vi "FT10_PXI-2565 Tester.vi"() -> ()   [LabVIEW 2024]
uses:
  <instrlib>/niSwitch/niSwitch.llb/niSwitch Topologies.ctl
  Controls/QMH Fundamentals - Message Cluster.ctl
  <instrlib>/niSwitch/niSwitch.llb/niSwitch Connect Channels (Single).vi
  <instrlib>/niSwitch/niSwitch.llb/niSwitch Disconnect Channels (Single).vi
panel:
  in  "Stop":bool
  out "instrument handle out":refnum<k15>
  out "error out":errorcluster {"code" format="%.0x"}
  in  "error in (no error)":errorcluster {"code" format="%.0x"}
  in  "reset device (boolean value)":bool=TRUE
  in  "simulate (boolean value)":bool
  in  "resource name":refnum<k15>="PXI1Slot7"
  in  "topology name":T1="2565/16-SPST"
  in  "Tab Control":enum32{"Manual", "Named"}(tab)
  in  "Channel 1":string
  in  "Channel 2":string
  in  "Disconnect - Manual":bool
  in  "Connect - Manual":bool
  in  "Enum":T2(ring)
  in  "Connect - Named":bool
  in  "Disconnect - Named":bool
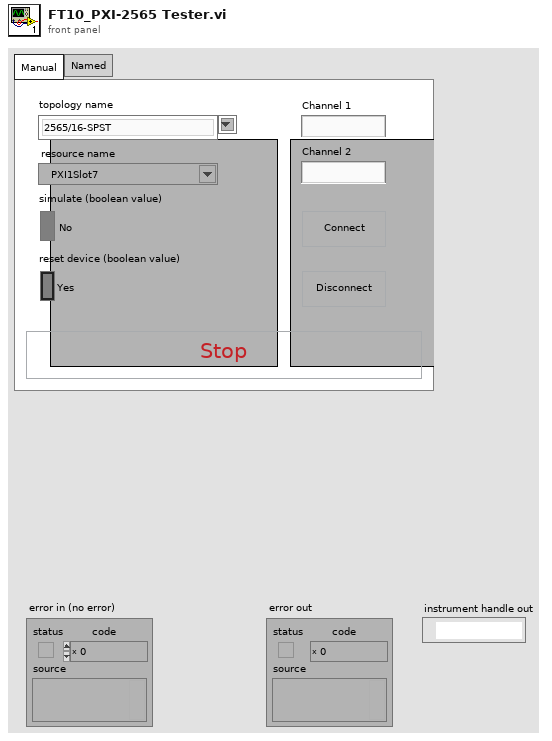
[diagram p1: front panel]
types:
  T1 = typedef "niSwitch Topologies.ctl" = string
  T2 = enum16{"Mono1 - Coag", "Mono1 - Cut", "Mono2 - Coag", "Mono2 - Cut", "Mono2 - Valleylab", "Mono2 - Spare", "Bipolar - Bipolar", "Advanced - Bipolar", "Advanced - Seal", "Advanced - Cut", "Advanced - Coag", "Advanced - Spare"}
  T3 = typedef "QMH Fundamentals - Message Cluster.ctl" = cluster{"Message":string, "Message Data":variant}
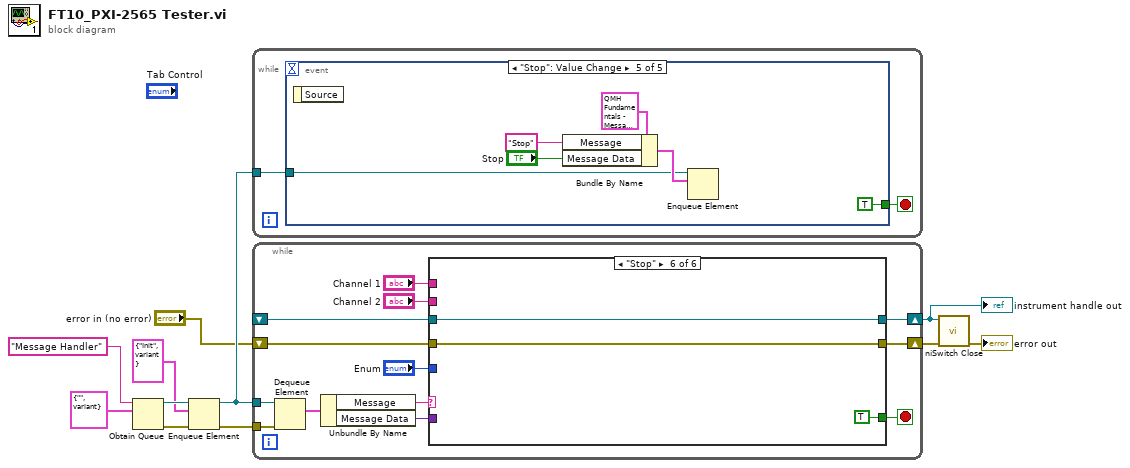
[diagram p0: block diagram]
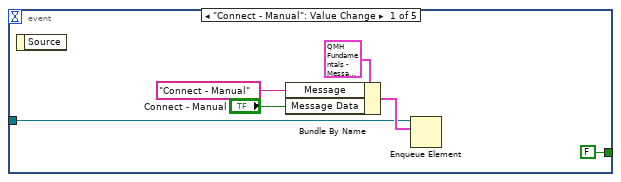
[diagram p2: hidden frame]
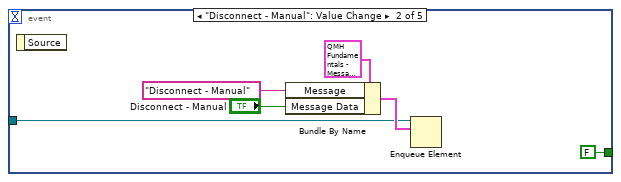
[diagram p3: hidden frame]
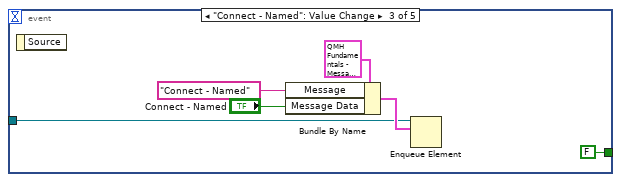
[diagram p4: hidden frame]
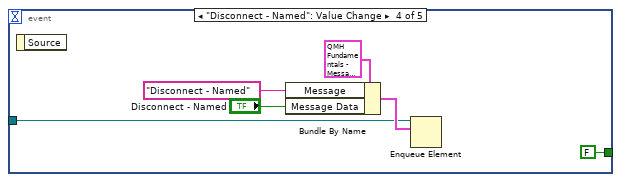
[diagram p5: hidden frame]
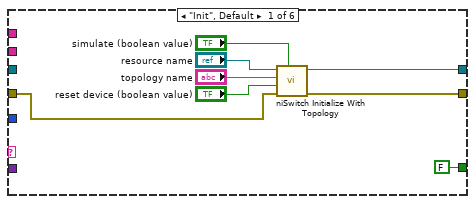
[diagram p6: hidden frame]
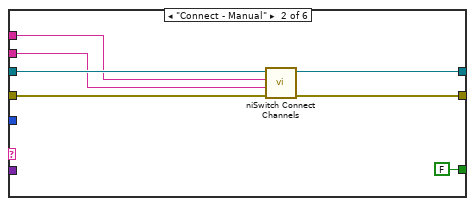
[diagram p7: hidden frame]
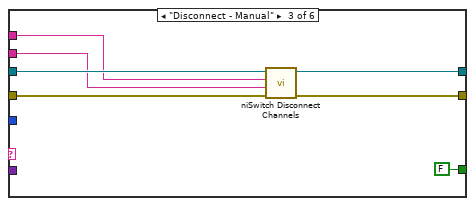
[diagram p8: hidden frame]
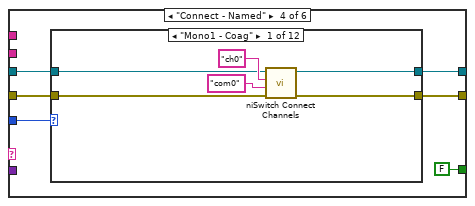
[diagram p9: hidden frame]
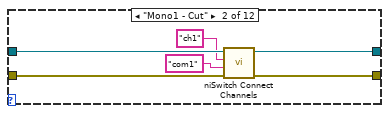
[diagram p10: hidden frame]
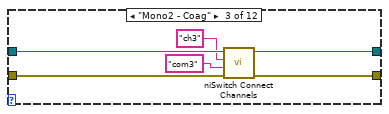
[diagram p11: hidden frame]
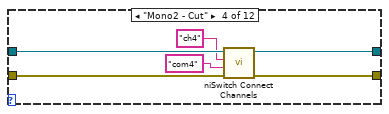
[diagram p12: hidden frame]
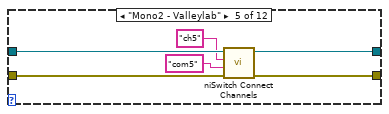
[diagram p13: hidden frame]
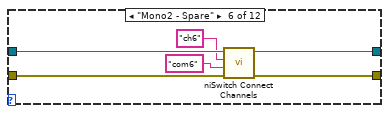
[diagram p14: hidden frame]
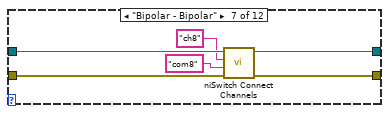
[diagram p15: hidden frame]
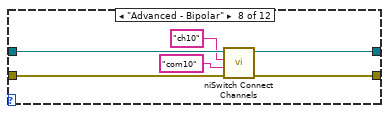
[diagram p16: hidden frame]
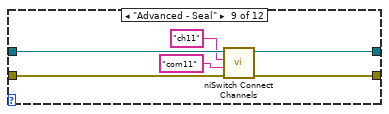
[diagram p17: hidden frame]
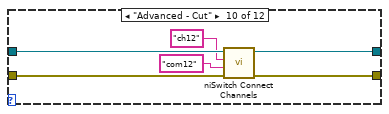
[diagram p18: hidden frame]
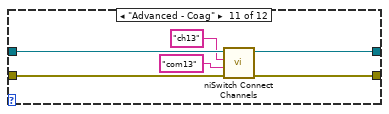
[diagram p19: hidden frame]
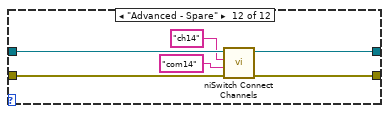
[diagram p20: hidden frame]
diagram:
  n1 = Obtain Queue(name (unnamed)="Message Handler", element data type=T3 {"Message"="", "Message Data"=variant} ("Message Cluster")) -> (queue out=w9:refnum<queue>, error out=w10:errorcluster)  [unwired: 3 in, 1 out]
  n2 = Enqueue Element(queue=w9, element=T3 {"Message"="Init", "Message Data"=variant}, error in (no error)=w10) -> (queue out=w5:refnum<queue>, error out=w6:errorcluster)  [unwired: 1 in, 1 out]
  n3 = while {
    tunnel: w5 -> [w13]
    stop <- w12 stop-if-true
    n4 = event shown="[4] \"Stop\": Value Change" {
      selector: _ -> [_ _ _ _ _]
      dyn-events: _ -> [_ _ _ _ _]
      timeout: _ -> [_ _ _ _ _]
      tunnel: w13 -> [w15 w22 w28 w34 w40]
      tunnel: [FALSE FALSE FALSE FALSE TRUE] -> w12
      event "Connect - Manual": Value Change {
        n5 = event-data() -> ()  [unwired: 1 in, 1 out]
        n6 = Bundle By Name(cluster=T3 {"Message"="Fornax Connect/Disconnect", "Message Data"=variant} ("element"), "Message"="Connect - Manual", "Message Data"="Connect - Manual") -> (w19:T3)
        n7 = Enqueue Element(queue=w15, element=w19) -> ()  [unwired: 2 in, 3 out]
      }
      event "Disconnect - Manual": Value Change {
        n8 = event-data() -> ()  [unwired: 1 in, 1 out]
        n9 = Bundle By Name(cluster=T3 {"Message"="Fornax Connect/Disconnect", "Message Data"=variant} ("element"), "Message"="Disconnect - Manual", "Message Data"="Disconnect - Manual") -> (w25:T3)
        n10 = Enqueue Element(queue=w22, element=w25) -> ()  [unwired: 2 in, 3 out]
      }
      event "Connect - Named": Value Change {
        n11 = event-data() -> ()  [unwired: 1 in, 1 out]
        n12 = Bundle By Name(cluster=T3 {"Message"="Fornax Connect/Disconnect", "Message Data"=variant} ("element"), "Message"="Connect - Named", "Message Data"="Connect - Named") -> (w31:T3)
        n13 = Enqueue Element(queue=w28, element=w31) -> ()  [unwired: 2 in, 3 out]
      }
      event "Disconnect - Named": Value Change {
        n14 = event-data() -> ()  [unwired: 1 in, 1 out]
        n15 = Bundle By Name(cluster=T3 {"Message"="Fornax Connect/Disconnect", "Message Data"=variant} ("element"), "Message"="Disconnect - Named", "Message Data"="Disconnect - Named") -> (w37:T3)
        n16 = Enqueue Element(queue=w34, element=w37) -> ()  [unwired: 2 in, 3 out]
      }
      event "Stop": Value Change {
        n17 = event-data() -> ()  [unwired: 1 in, 1 out]
        n18 = Bundle By Name(cluster=T3 {"Message"="Fornax Connect/Disconnect", "Message Data"=variant} ("element"), "Message"="Stop", "Message Data"="Stop") -> (w43:T3)
        n19 = Enqueue Element(queue=w40, element=w43) -> ()  [unwired: 2 in, 3 out]
      }
    }
  }
  n20 = while {
    tunnel: w5 -> [w55]
    tunnel: w6 -> [w54]
    shift-right: [w51] -> w3
    shift-left: _ -> [w50]
    shift-right: [w47] -> w2
    shift-left: "error in (no error)" -> [w46]
    stop <- w44 stop-if-true
    n21 = Dequeue Element(queue=w55, error in (no error)=w54) -> (element=w56:T3)  [unwired: 1 in, 3 out]
    n22 = Unbundle By Name(w56) -> ("Message"=w53:string, "Message Data"=w52:variant)
    n23 = case shown="\"Stop\"" w53 {
      tunnel: w52 -> [_ _ _ _ _ _]
      tunnel: [w60 w68 w73 w82 w160 w237] -> w51
      tunnel: w50 -> [_ w71 w78 w84 w162 w237]
      tunnel: "Channel 1" -> [_ w70 w77 _ _ _]
      tunnel: "Channel 2" -> [_ w69 w76 _ _ _]
      tunnel: [w59 w66 w74 w81 w159 w236] -> w47
      tunnel: w46 -> [w58 w67 w75 w83 w161 w236]
      tunnel: "Enum" -> [_ _ _ w80 w158 _]
      tunnel: [FALSE FALSE FALSE FALSE FALSE TRUE] -> w44
      frame "Init", Default {
        n24 = call <instrlib>:"niSwitch Initialize With Topology.vi"("simulate (boolean value)"="simulate (boolean value)", "error in (no error)"=w58, "reset device (boolean value)"="reset device (boolean value)", "topology name"="topology name", "resource name"="resource name") -> ("error out"=w59:errorcluster, "instrument handle out"=w60:refnum<k15>)  [unwired: 5 in]
      }
      frame "Connect - Manual" {
        n25 = call-poly <instrlib>:"niSwitch Connect Channels.vi"("error in (no error)"=w67, "channel 2"=w69, "channel 1"=w70, "instrument handle"=w71) -> ("error out"=w66:errorcluster, "instrument handle out"=w68:refnum<k15>)  [unwired: 6 in]
      }
      frame "Disconnect - Manual" {
        n26 = call-poly <instrlib>:"niSwitch Disconnect Channels.vi"("error in (no error)"=w75, "channel 2"=w76, "channel 1"=w77, "instrument handle"=w78) -> ("error out"=w74:errorcluster, "instrument handle out"=w73:refnum<k15>)  [unwired: 6 in]
      }
      frame "Connect - Named" {
        n27 = case shown="\"Mono1 - Coag\"" w80 {
          tunnel: w84 -> [w88 w96 w102 w108 w114 w120 w126 w132 w138 w144 w150 w156]
          tunnel: w83 -> [w87 w95 w101 w107 w113 w119 w125 w131 w137 w143 w149 w155]
          tunnel: [w86 w94 w100 w106 w112 w118 w124 w130 w136 w142 w148 w154] -> w82
          tunnel: [w85 w93 w99 w105 w111 w117 w123 w129 w135 w141 w147 w153] -> w81
          frame "Mono1 - Coag" {
            n28 = call-poly <instrlib>:"niSwitch Connect Channels.vi"("error in (no error)"=w87, "channel 2"="com0", "channel 1"="ch0", "instrument handle"=w88) -> ("error out"=w85:errorcluster, "instrument handle out"=w86:refnum<k15>)  [unwired: 6 in]
          }
          frame "Mono1 - Cut" {
            n29 = call-poly <instrlib>:"niSwitch Connect Channels.vi"("error in (no error)"=w95, "channel 2"="com1", "channel 1"="ch1", "instrument handle"=w96) -> ("error out"=w93:errorcluster, "instrument handle out"=w94:refnum<k15>)  [unwired: 6 in]
          }
          frame "Mono2 - Coag" {
            n30 = call-poly <instrlib>:"niSwitch Connect Channels.vi"("error in (no error)"=w101, "channel 2"="com3", "channel 1"="ch3", "instrument handle"=w102) -> ("error out"=w99:errorcluster, "instrument handle out"=w100:refnum<k15>)  [unwired: 6 in]
          }
          frame "Mono2 - Cut" {
            n31 = call-poly <instrlib>:"niSwitch Connect Channels.vi"("error in (no error)"=w107, "channel 2"="com4", "channel 1"="ch4", "instrument handle"=w108) -> ("error out"=w105:errorcluster, "instrument handle out"=w106:refnum<k15>)  [unwired: 6 in]
          }
          frame "Mono2 - Valleylab" {
            n32 = call-poly <instrlib>:"niSwitch Connect Channels.vi"("error in (no error)"=w113, "channel 2"="com5", "channel 1"="ch5", "instrument handle"=w114) -> ("error out"=w111:errorcluster, "instrument handle out"=w112:refnum<k15>)  [unwired: 6 in]
          }
          frame "Mono2 - Spare" {
            n33 = call-poly <instrlib>:"niSwitch Connect Channels.vi"("error in (no error)"=w119, "channel 2"="com6", "channel 1"="ch6", "instrument handle"=w120) -> ("error out"=w117:errorcluster, "instrument handle out"=w118:refnum<k15>)  [unwired: 6 in]
          }
          frame "Bipolar - Bipolar" {
            n34 = call-poly <instrlib>:"niSwitch Connect Channels.vi"("error in (no error)"=w125, "channel 2"="com8", "channel 1"="ch8", "instrument handle"=w126) -> ("error out"=w123:errorcluster, "instrument handle out"=w124:refnum<k15>)  [unwired: 6 in]
          }
          frame "Advanced - Bipolar" {
            n35 = call-poly <instrlib>:"niSwitch Connect Channels.vi"("error in (no error)"=w131, "channel 2"="com10", "channel 1"="ch10", "instrument handle"=w132) -> ("error out"=w129:errorcluster, "instrument handle out"=w130:refnum<k15>)  [unwired: 6 in]
          }
          frame "Advanced - Seal" {
            n36 = call-poly <instrlib>:"niSwitch Connect Channels.vi"("error in (no error)"=w137, "channel 2"="com11", "channel 1"="ch11", "instrument handle"=w138) -> ("error out"=w135:errorcluster, "instrument handle out"=w136:refnum<k15>)  [unwired: 6 in]
          }
          frame "Advanced - Cut" {
            n37 = call-poly <instrlib>:"niSwitch Connect Channels.vi"("error in (no error)"=w143, "channel 2"="com12", "channel 1"="ch12", "instrument handle"=w144) -> ("error out"=w141:errorcluster, "instrument handle out"=w142:refnum<k15>)  [unwired: 6 in]
          }
          frame "Advanced - Coag" {
            n38 = call-poly <instrlib>:"niSwitch Connect Channels.vi"("error in (no error)"=w149, "channel 2"="com13", "channel 1"="ch13", "instrument handle"=w150) -> ("error out"=w147:errorcluster, "instrument handle out"=w148:refnum<k15>)  [unwired: 6 in]
          }
          frame "Advanced - Spare" {
            n39 = call-poly <instrlib>:"niSwitch Connect Channels.vi"("error in (no error)"=w155, "channel 2"="com14", "channel 1"="ch14", "instrument handle"=w156) -> ("error out"=w153:errorcluster, "instrument handle out"=w154:refnum<k15>)  [unwired: 6 in]
          }
        }
      }
      frame "Disconnect - Named" {
        n40 = case shown="\"Mono1 - Coag\"" w158 {
          tunnel: w162 -> [w166 w174 w180 w186 w192 w198 w204 w210 w216 w222 w228 w234]
          tunnel: w161 -> [w165 w173 w179 w185 w191 w197 w203 w209 w215 w221 w227 w233]
          tunnel: [w164 w172 w178 w184 w190 w196 w202 w208 w214 w220 w226 w232] -> w160
          tunnel: [w163 w171 w177 w183 w189 w195 w201 w207 w213 w219 w225 w231] -> w159
          frame "Mono1 - Coag" {
            n41 = call-poly <instrlib>:"niSwitch Disconnect Channels.vi"("error in (no error)"=w165, "channel 2"="com0", "channel 1"="ch0", "instrument handle"=w166) -> ("error out"=w163:errorcluster, "instrument handle out"=w164:refnum<k15>)  [unwired: 6 in]
          }
          frame "Mono1 - Cut" {
            n42 = call-poly <instrlib>:"niSwitch Disconnect Channels.vi"("error in (no error)"=w173, "channel 2"="com1", "channel 1"="ch1", "instrument handle"=w174) -> ("error out"=w171:errorcluster, "instrument handle out"=w172:refnum<k15>)  [unwired: 6 in]
          }
          frame "Mono2 - Coag" {
            n43 = call-poly <instrlib>:"niSwitch Disconnect Channels.vi"("error in (no error)"=w179, "channel 2"="com3", "channel 1"="ch3", "instrument handle"=w180) -> ("error out"=w177:errorcluster, "instrument handle out"=w178:refnum<k15>)  [unwired: 6 in]
          }
          frame "Mono2 - Cut" {
            n44 = call-poly <instrlib>:"niSwitch Disconnect Channels.vi"("error in (no error)"=w185, "channel 2"="com4", "channel 1"="ch4", "instrument handle"=w186) -> ("error out"=w183:errorcluster, "instrument handle out"=w184:refnum<k15>)  [unwired: 6 in]
          }
          frame "Mono2 - Valleylab" {
            n45 = call-poly <instrlib>:"niSwitch Disconnect Channels.vi"("error in (no error)"=w191, "channel 2"="com5", "channel 1"="ch5", "instrument handle"=w192) -> ("error out"=w189:errorcluster, "instrument handle out"=w190:refnum<k15>)  [unwired: 6 in]
          }
          frame "Mono2 - Spare" {
            n46 = call-poly <instrlib>:"niSwitch Disconnect Channels.vi"("error in (no error)"=w197, "channel 2"="com6", "channel 1"="ch6", "instrument handle"=w198) -> ("error out"=w195:errorcluster, "instrument handle out"=w196:refnum<k15>)  [unwired: 6 in]
          }
          frame "Bipolar - Bipolar" {
            n47 = call-poly <instrlib>:"niSwitch Disconnect Channels.vi"("error in (no error)"=w203, "channel 2"="com8", "channel 1"="ch8", "instrument handle"=w204) -> ("error out"=w201:errorcluster, "instrument handle out"=w202:refnum<k15>)  [unwired: 6 in]
          }
          frame "Advanced - Bipolar" {
            n48 = call-poly <instrlib>:"niSwitch Disconnect Channels.vi"("error in (no error)"=w209, "channel 2"="com10", "channel 1"="ch10", "instrument handle"=w210) -> ("error out"=w207:errorcluster, "instrument handle out"=w208:refnum<k15>)  [unwired: 6 in]
          }
          frame "Advanced - Seal" {
            n49 = call-poly <instrlib>:"niSwitch Disconnect Channels.vi"("error in (no error)"=w215, "channel 2"="com11", "channel 1"="ch11", "instrument handle"=w216) -> ("error out"=w213:errorcluster, "instrument handle out"=w214:refnum<k15>)  [unwired: 6 in]
          }
          frame "Advanced - Cut" {
            n50 = call-poly <instrlib>:"niSwitch Disconnect Channels.vi"("error in (no error)"=w221, "channel 2"="com12", "channel 1"="ch12", "instrument handle"=w222) -> ("error out"=w219:errorcluster, "instrument handle out"=w220:refnum<k15>)  [unwired: 6 in]
          }
          frame "Advanced - Coag" {
            n51 = call-poly <instrlib>:"niSwitch Disconnect Channels.vi"("error in (no error)"=w227, "channel 2"="com13", "channel 1"="ch13", "instrument handle"=w228) -> ("error out"=w225:errorcluster, "instrument handle out"=w226:refnum<k15>)  [unwired: 6 in]
          }
          frame "Advanced - Spare" {
            n52 = call-poly <instrlib>:"niSwitch Disconnect Channels.vi"("error in (no error)"=w233, "channel 2"="com14", "channel 1"="ch14", "instrument handle"=w234) -> ("error out"=w231:errorcluster, "instrument handle out"=w232:refnum<k15>)  [unwired: 6 in]
          }
        }
      }
      frame "Stop" {
      }
    }
  }
  "instrument handle out" <- w3
  n53 = call <instrlib>:"niSwitch Close.vi"("error in (no error)"=w2, "instrument handle"=w3) -> ("error out"=→"error out":errorcluster)  [unwired: 9 in]
